vi "Init.vi"(8 "error in":errorcluster, 10 "<JSON> Const Action Data":string, 11 "Perform Action Red-y Read Write Strategy in":refnum<class "Perform Action Red-y Read Write Strategy.lvclass">) -> (0 "error out":errorcluster, 3 "Perform Action Red-y Read Write Strategy out":refnum<class "Perform Action Red-y Read Write Strategy.lvclass">)   [LabVIEW 2024, in "Perform Action Red-y Read Write Strategy.lvclass"]
uses:
  Perform Action Red-y Read Write Strategy.lvclass
  Perform Action Red-y Read Write Strategy.lvclass/Perform Action Red-y Read Write Strategy.ctl
  2a6defca-0460-46ea-9309-12a78dfa7b98.vi
  <vilib>/JDP Science/JSONtext/JSON text to Variant.vi
  <vilib>/JDP Science/JSONtext/LVClass Serializer/JSONtext LVClass Serializer.lvclass
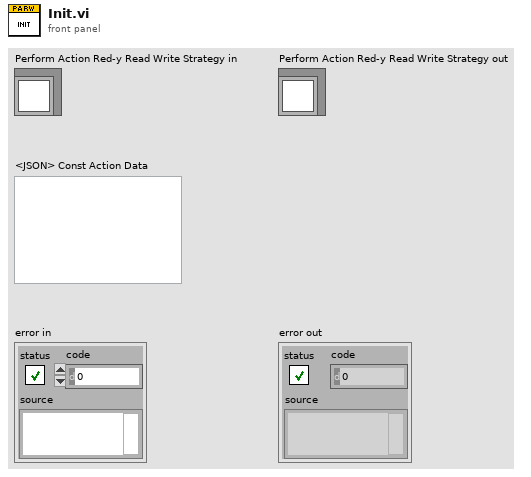
[diagram p1: front panel]
types:
  T1 = cluster{"Action":enum16{"Write", "Read"}, "Register":string, "Type":string}
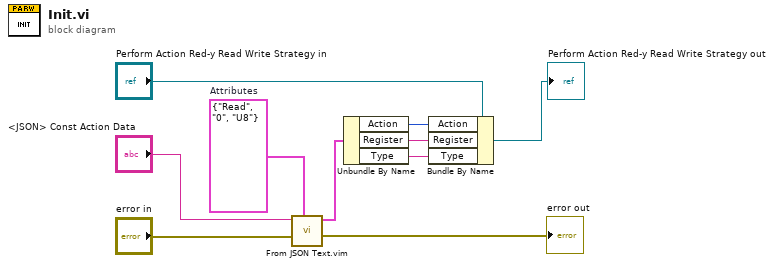
[diagram p0: block diagram]
diagram:
  w8 = T1 {"Action"=enum."Read", "Register"="0", "Type"="U8"}  # Attributes
  n1 = call "From JSON Text.vim"("Data Type and Default Value"=w8, "error in (no error)"="error in", "JSON"="<JSON> Const Action Data") -> ("error out"=→"error out":errorcluster, "Data out"=w4:T1)  [unwired: 7 in]
  n2 = Unbundle By Name(w4) -> ("Action"=w3:enum16{"Write", "Read"}, "Register"=w2:string, "Type"=w1:string)
  n3 = Bundle By Name(cluster="Perform Action Red-y Read Write Strategy in", "Action"=w3, "Register"=w2, "Type"=w1) -> (→"Perform Action Red-y Read Write Strategy out":refnum<class "Perform Action Red-y Read Write Strategy.lvclass">)
